vi "Test1.vi"() -> ()   [LabVIEW 2016]
panel:
  out "Error Out":errorcluster
  in  "Error In":errorcluster
  in  "stop":bool
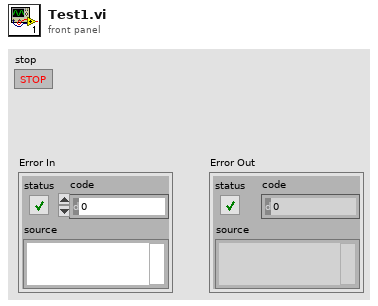
[diagram p1: front panel]
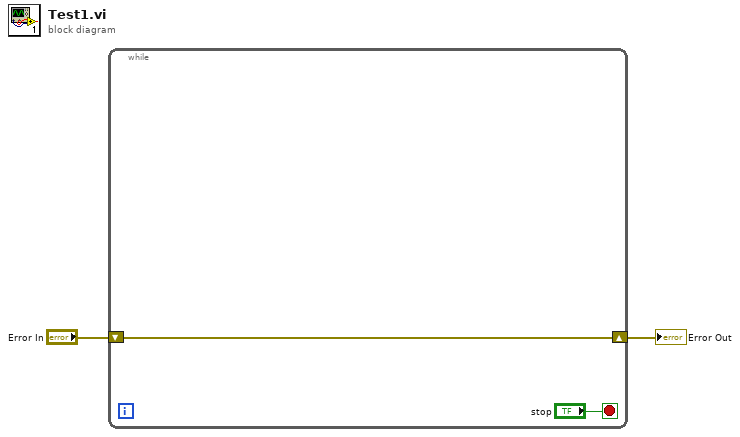
[diagram p0: block diagram]
diagram:
  n1 = while {
    shift-right: [w3] -> w1
    shift-left: "Error In" -> [w3]
    stop <- "stop" stop-if-true
  }
  "Error Out" <- w1
